vi "H5Pset_btree_ratios.vi"(5 "Middle":dbl=0.5 min=0.0 max=1.0, 6 "error in (no error)":errorcluster, 7 "Right":dbl=0.5 min=0.0 max=1.0, 8 "Left":dbl=0.5 min=0.0 max=1.0, 9 "HDF5 Property Ref":T1) -> (0 "error out":errorcluster, 3 "HDF5 Ref out":T1)   [LabVIEW 2017]
doc: "Sets B-tree split ratios for a dataset transfer property list."
uses:
  <vilib>/UPVI/lvhdf5/library.llb/HDF5 Ref.ctl
  <vilib>/UPVI/lvhdf5/hdf5.dll
panel:
  # "LVHDF5 Toolkit\nCopyright (c) 2005-2013 by Jason D. Sommerville\nCopyright (c) 2014 by UPVI, LLC.\n\nThis use and distribution of this file is governed by the terms found in \nLICENSE.txt distributed with this toolkit and installed at\n <user.lib>\\_lvhdf5\\LICENSE.txt"
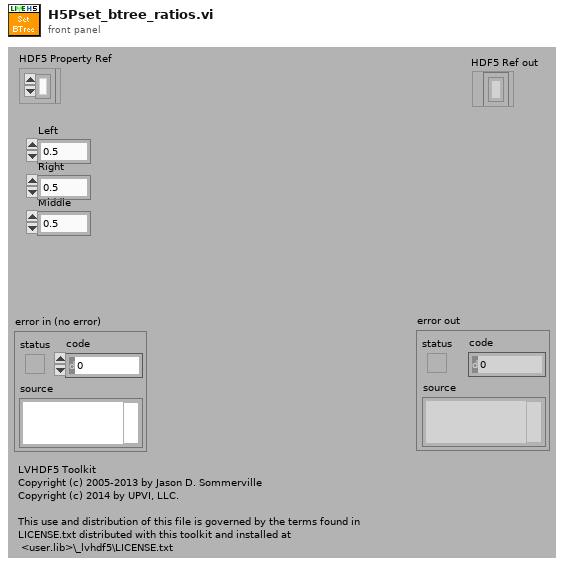
[diagram p1: front panel]
types:
  T1 = typedef "HDF5 Ref.ctl" = refnum<k1>
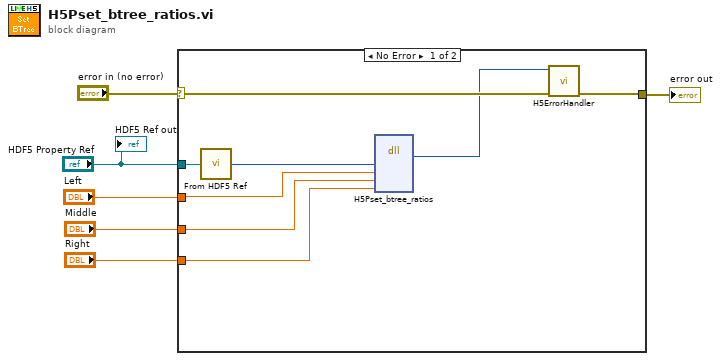
[diagram p0: block diagram]
diagram:
  n1 = case shown="No Error" "error in (no error)" {
    selector: "error in (no error)" -> [w14 w15]
    tunnel: [w13 w15] -> w5
    tunnel: "HDF5 Property Ref" -> [w11 _]
    tunnel: "Left" -> [w9 _]
    tunnel: "Middle" -> [w8 _]
    tunnel: "Right" -> [w7 _]
    frame No Error {
      n2 = call <vilib>:"From HDF5 Ref.vi"("HDF5 Ref"=w11) -> ("I32"=w10:i32)
      n3 = dll-call lib="C:/Program Files/National Instruments/LabVIEW 2017/vi.lib/UPVI/lvhdf5/hdf5.dll" fn="H5Pset_btree_ratios"("plist_id"=w10, "left"=w9, "middle"=w8, "right"=w7) -> (w12:i32)  [unwired: 7 in, 2 out]
      n4 = call <vilib>:"H5ErrorHandler.vi"("error in (no error)"=w14, "herr_t"=w12) -> ("error out"=w13:errorcluster)  [unwired: 3 in, 4 out]
    }
    frame Error {
    }
  }
  "error out" <- w5
  "HDF5 Ref out" <- "HDF5 Property Ref"
